vi "DHE_DRV_support_read_actual_inttime.vi"(5 "support rit?":bool, 11 "error in (no error)":errorcluster) -> (8 "return value":i32, 15 "error out":errorcluster)   [LabVIEW 2016]
doc: "This VI closes the I/O interface with the instrument."
uses:
  c/lib/libarcDHE.so
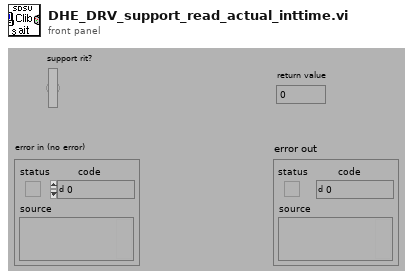
[diagram p1: front panel]
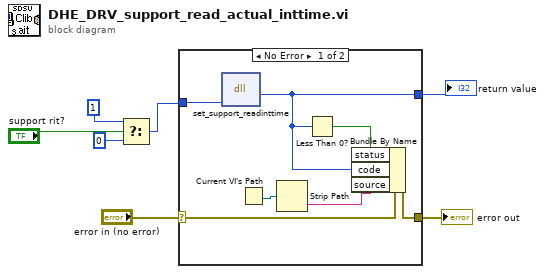
[diagram p0: block diagram]
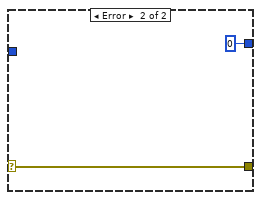
[diagram p2: hidden frame]
diagram:
  n1 = Select(t=1, s="support rit?", f=0) -> (s? t:f=w1:i32)
  n2 = case shown="No Error" "error in (no error)" {
    selector: "error in (no error)" -> [w8 w15]
    tunnel: w1 -> [w14 _]
    tunnel: [w12 0] -> w7
    tunnel: [w9 w15] -> w6
    frame No Error {
      n3 = dll-call lib="home/simager/panview/PAN/Modules/SDSU/private/c/lib/libarcDHE.so" fn="set_support_readinttime" label="support abort read"("srit"=w14) -> ("return type"=w12:i32)  [unwired: 3 in, 3 out]
      n4 = Current VI's Path() -> (path=w11:path)
      n5 = Strip Path(path=w11) -> (name=w10:string)  [unwired: 1 out]
      n6 = Less Than 0?(x=w12) -> (x < 0?=w13:bool)
      n7 = Bundle By Name(cluster=w8, "status"=w13, "code"=w12, "source"=w10) -> (w9:errorcluster)
    }
    frame Error {
    }
  }
  "error out" <- w6
  "return value" <- w7
